vi "ReadExEventFINAL_working.vi"() -> ()   [LabVIEW 2015]
uses:
  GPS_Driver_Global.vi
panel:
  in  "Path to FITS Header File":path=path "C:/Users/Public/Documents/SI Image SGL II -/Other Parameters.txt"
  out "# Entries After":i16
  in  "# Entries Before":i16
  out "Close Min":u32
  out "Close Maj":u32
  out "Open Min":u32
  out "Open Maj":u32
  out "error out":errorcluster
  in  "error in (no error)":errorcluster
  # "Major UNIX Time:"
  # "Minor UNIX Time:"
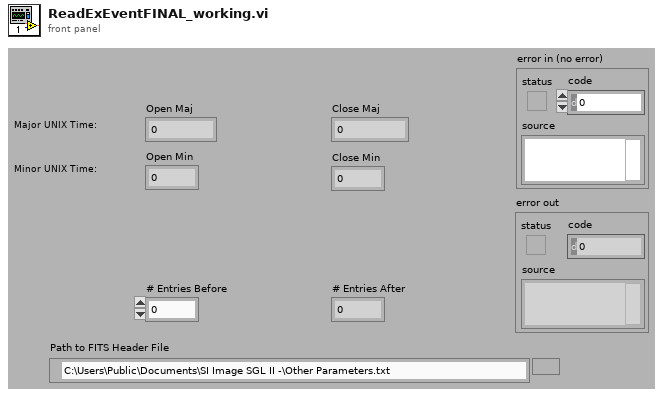
[diagram p1: front panel]
types:
  T1 = cluster{"Close":cluster{"Time":string, "Error":string}, "Open":cluster{"Time":string, "Error":string}}
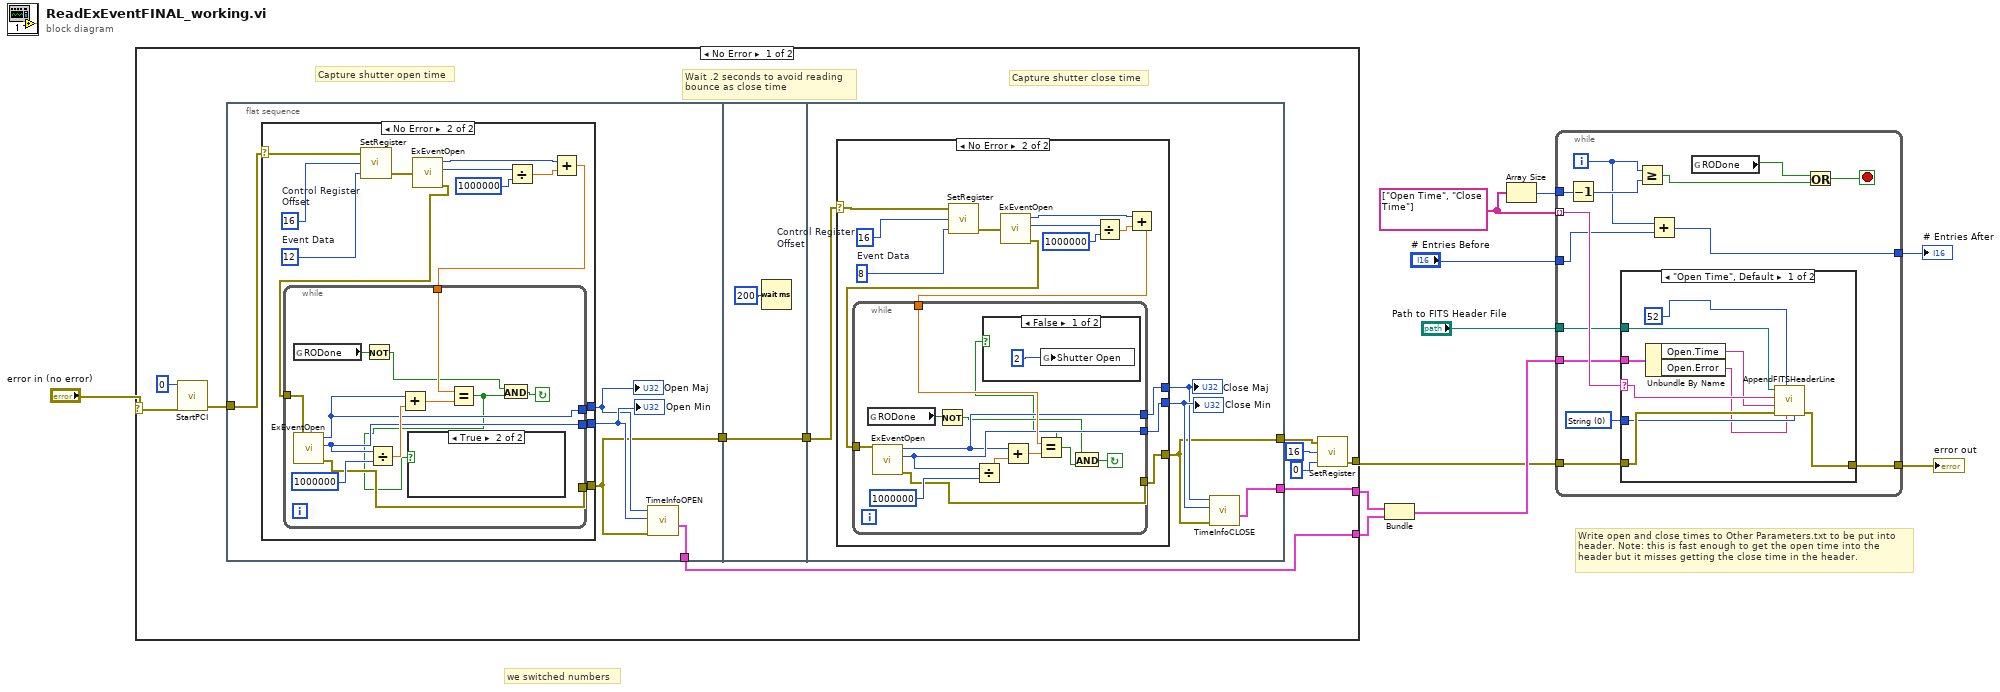
[diagram p0: block diagram]
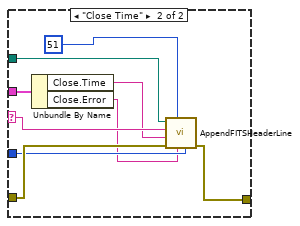
[diagram p2: hidden frame]
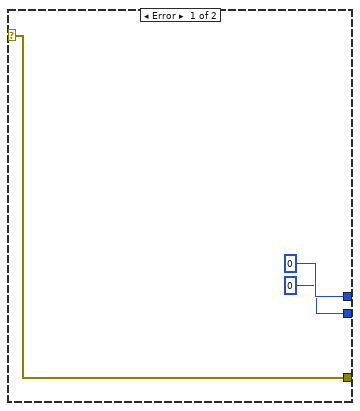
[diagram p3: hidden frame]
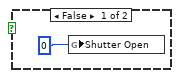
[diagram p4: hidden frame]
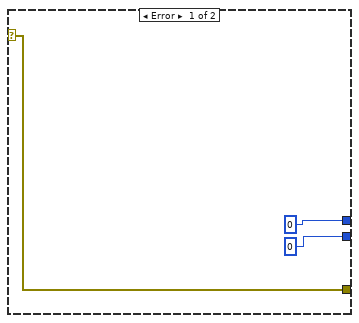
[diagram p5: hidden frame]
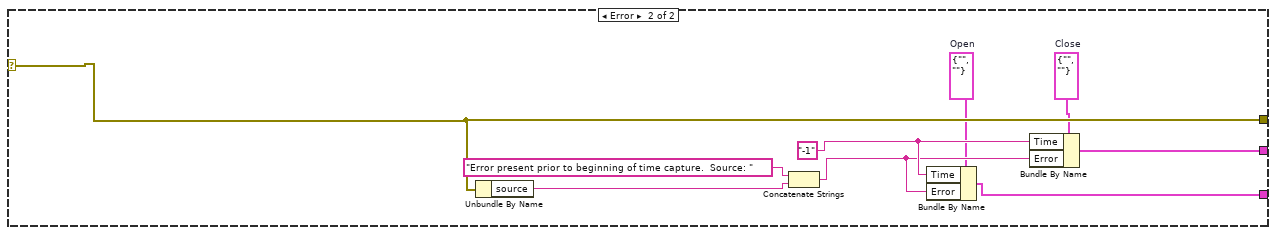
[diagram p7: hidden frame]
diagram:
  w11 = string[] ["Open Time", "Close Time"]
  # "we switched numbers"
  # "Write open and close times to Other Parameters.txt to be put into\nheader. Note: this is fast enough to get the open time into the \nheader but it misses getting the close time in the header."
  n1 = case shown="No Error" "error in (no error)" {
    selector: "error in (no error)" -> [w18 w101]
    tunnel: [w19 w101] -> w6
    tunnel: [w16 w93] -> w7
    tunnel: [w15 w97] -> w8
    frame No Error {
      # "Capture shutter close time"
      # "Wait .2 seconds to avoid reading \nbounce as close time"
      # "Capture shutter open time"
      n2 = call "StartPCI.vi"("error in (no error)"=w18, "Device Number"=0) -> ("error out"=w17:errorcluster)  [unwired: 4 in]
      n3 = flat-sequence {
        tunnel: w17 -> [w25]
        tunnel: [w24] -> w16
        tunnel: [w23] -> w13
        tunnel: [w58] -> w14
        tunnel: w13 -> [w58]
        tunnel: [w61] -> w15
        tunnel: w14 -> [w60]
        tunnel: [w59] -> w12
        frame #0 {
          n4 = case shown="No Error" w25 {
            selector: w25 -> [w28 w31]
            tunnel: [0 w41] -> w27
            tunnel: [w28 w40] -> w23
            tunnel: [0 w39] -> w26
            frame Error {
            }
            frame No Error {
              w42 = 12  # Event Data
              w43 = 16  # Control Register Offset
              n5 = call "SetRegister.vi"("Data"=w42, "Offset"=w43, "error in (no error)"=w31) -> ("error out"=w38:errorcluster)  [unwired: 2 in]
              n6 = call "ExEventOpen.vi"("error in (no error)"=w38) -> ("Major Time"=w34:u32, "Minor Time"=w37:u32, "error out"=w35:errorcluster)  [unwired: 1 in]
              n7 = Divide(x=w37, y=1000000) -> (x/y=w33:dbl)
              n8 = Add(x=w34, y=w33) -> (x+y=w32:dbl)
              n9 = while {
                tunnel: w35 -> [w55]
                tunnel: w32 -> [w54]
                tunnel: [w51] -> w40
                tunnel: [w49] -> w39
                tunnel: [w48] -> w41
                stop <- w47 continue-if-true
                n10 = global read "GPS_Driver_Global.vi" "RODone"() -> (w45:bool)
                n11 = call "ExEventOpen.vi"("error in (no error)"=w55) -> ("Major Time"=w49:u32, "Minor Time"=w48:u32, "error out"=w51:errorcluster)  [unwired: 1 in]
                n12 = Not(x=w45) -> (.not. x?=w46:bool)
                n13 = Divide(x=w48, y=1000000) -> (x/y=w53:dbl)
                n14 = Add(x=w49, y=w53) -> (x+y=w50:dbl)
                n15 = Equal?(x=w54, y=w50) -> (x = y?=w44:bool)
                n16 = case shown="True" w44 {
                  frame False {
                    n17 = global write "GPS_Driver_Global.vi" "Shutter Open"(0) -> ()
                  }
                  frame True {
                  }
                }
                n18 = And(x=w46, y=w44) -> (x .and. y?=w47:bool)
              }
            }
          }
          "Open Min" <- w27
          "Open Maj" <- w26
          n19 = call "TimeInfoOPEN.vi"("error in (no error)"=w23, "Minor Time"=w27, "Major Time"=w26) -> ("Open"=w24:cluster{"Time":string, "Error":string})  [unwired: 6 in, 1 out]
        }
        frame #1 {
          n20 = Wait (ms)(milliseconds to wait=200) -> ()  [unwired: 1 out]
        }
        frame #2 {
          n21 = case shown="No Error" w60 {
            selector: w60 -> [w64 w67]
            tunnel: [0 w77] -> w63
            tunnel: [w64 w76] -> w59
            tunnel: [0 w75] -> w62
            frame Error {
            }
            frame No Error {
              w78 = 8  # Event Data
              w79 = 16  # Control Register Offset
              n22 = call "SetRegister.vi"("Data"=w78, "Offset"=w79, "error in (no error)"=w67) -> ("error out"=w74:errorcluster)  [unwired: 2 in]
              n23 = call "ExEventOpen.vi"("error in (no error)"=w74) -> ("Major Time"=w70:u32, "Minor Time"=w73:u32, "error out"=w71:errorcluster)  [unwired: 1 in]
              n24 = Divide(x=w73, y=1000000) -> (x/y=w69:dbl)
              n25 = Add(x=w70, y=w69) -> (x+y=w68:dbl)
              n26 = while {
                tunnel: w71 -> [w91]
                tunnel: w68 -> [w90]
                tunnel: [w87] -> w76
                tunnel: [w84] -> w75
                tunnel: [w86] -> w77
                stop <- w83 continue-if-true
                n27 = global read "GPS_Driver_Global.vi" "RODone"() -> (w81:bool)
                n28 = call "ExEventOpen.vi"("error in (no error)"=w91) -> ("Major Time"=w84:u32, "Minor Time"=w86:u32, "error out"=w87:errorcluster)  [unwired: 1 in]
                n29 = Not(x=w81) -> (.not. x?=w82:bool)
                n30 = Divide(x=w86, y=1000000) -> (x/y=w89:dbl)
                n31 = Add(x=w84, y=w89) -> (x+y=w85:dbl)
                n32 = Equal?(x=w90, y=w85) -> (x = y?=w80:bool)
                n33 = case shown="False" w80 {
                  frame False {
                    n34 = global write "GPS_Driver_Global.vi" "Shutter Open"(2) -> ()
                  }
                  frame True {
                  }
                }
                n35 = And(x=w82, y=w80) -> (x .and. y?=w83:bool)
              }
            }
          }
          "Close Maj" <- w62
          "Close Min" <- w63
          n36 = call "TimeInfoCLOSE.vi"("error in (no error)"=w59, "Minor Time"=w63, "Major Time"=w62) -> ("Close"=w61:cluster{"Time":string, "Error":string})  [unwired: 7 in]
        }
      }
      n37 = call "SetRegister.vi"("Data"=0, "Offset"=16, "error in (no error)"=w12) -> ("error out"=w19:errorcluster)  [unwired: 2 in]
    }
    frame Error {
      w98 = cluster{"Time":string, "Error":string} {"Time"="", "Error"=""}  # Close
      w94 = cluster{"Time":string, "Error":string} {"Time"="", "Error"=""}  # Open
      w96 = "-1"
      n38 = Unbundle By Name(w101) -> ("source"=w99:string)
      n39 = Concatenate Strings("Error present prior to beginning of time capture.  Source: ", w99) -> (w95:string)
      n40 = Bundle By Name(cluster=w94, "Time"=w96, "Error"=w95) -> (w93:cluster{"Time":string, "Error":string})
      n41 = Bundle By Name(cluster=w98, "Time"=w96, "Error"=w95) -> (w97:cluster{"Time":string, "Error":string})
    }
  }
  n42 = Bundle("Close"=w8, "Open"=w7) -> (w10:T1)  [unwired: 1 in]
  n43 = Array Size(array=w11) -> (size(s)=w4:i32)
  n44 = while {
    tunnel: w6 -> [w115]
    tunnel: w11 -> [w113] mode=indexing
    tunnel: w4 -> [w112]
    tunnel: "# Entries Before" -> [w110]
    tunnel: w10 -> [w108]
    tunnel: "Path to FITS Header File" -> [w107]
    tunnel: [w106] -> w9
    tunnel: [w102] -> w2
    i -> [w109]
    stop <- w104 stop-if-true
    w111 = u16 0 items=["String", "Numeric", "Boolean"]
    n45 = Decrement(x=w112) -> (x-1=w114:i32)
    n46 = case shown="\"Open Time\", Default" w113 {
      selector: w113 -> [w122 w132]
      tunnel: w115 -> [w124 w133]
      tunnel: w111 -> [w123 w131]
      tunnel: w108 -> [w119 w128]
      tunnel: w107 -> [w121 w129]
      tunnel: [w120 w130] -> w106
      frame "Open Time", Default {
        n47 = Unbundle By Name(w119) -> ("Open.Time"=w118:string, "Open.Error"=w117:string)
        n48 = call "AppendFITSHeaderLine.vi"("Entry Type"=w123, "Comment"=w117, "Entry #"=52, "error in (no error)"=w124, "Element Value"=w118, "Element Name"=w122, "file path (dialog if empty)"=w121) -> ("error out"=w120:errorcluster)  [unwired: 3 in]
      }
      frame "Close Time" {
        n49 = Unbundle By Name(w128) -> ("Close.Time"=w127:string, "Close.Error"=w126:string)
        n50 = call "AppendFITSHeaderLine.vi"("Entry Type"=w131, "Comment"=w126, "Entry #"=51, "error in (no error)"=w133, "Element Value"=w127, "Element Name"=w132, "file path (dialog if empty)"=w129) -> ("error out"=w130:errorcluster)  [unwired: 3 in]
      }
    }
    n51 = Greater Or Equal?(x=w109, y=w114) -> (x >= y?=w105:bool)
    n52 = Add(x=w109, y=w110) -> (x+y=w102:i32)
    n53 = global read "GPS_Driver_Global.vi" "RODone"() -> (w103:bool)
    n54 = Or(x=w103, y=w105) -> (x .or. y?=w104:bool)
  }
  "error out" <- w9
  "# Entries After" <- w2
